vi "335 set Temp(SubVI).vi"(6 "Input (0:A)":u16(ring)=1 items=["A", "B"], 7 "Output (1:1)":u16(ring)=1 items=["1"=1, "2"=2], 8 "error in (no error)":errorcluster, 9 "Rate":dbl, 10 "Temperature":dbl, 11 "VISA Refnum in":refnum<visa-resource-name>) -> (0 "error out":errorcluster, 3 "VISA resource name out":refnum<visa-resource-name>)   [LabVIEW 2019, in "SubVI.lvlib"]
uses:
  SubVI.lvlib
  lib/Lake Shore 335/Lake Shore 335.lvlib
panel:
  out "Sensor Data 2":dbl format="%.4f"
  out "Sensor Data":dbl format="%.4f"
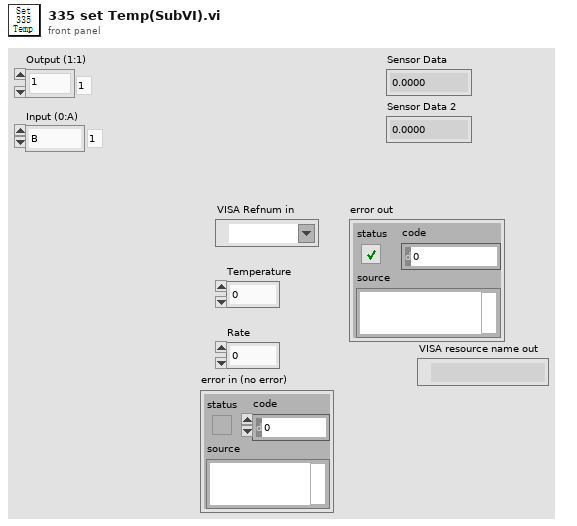
[diagram p1: front panel]
types:
  T1 = typedef "Semaphore RefNum" = refnum<k1>
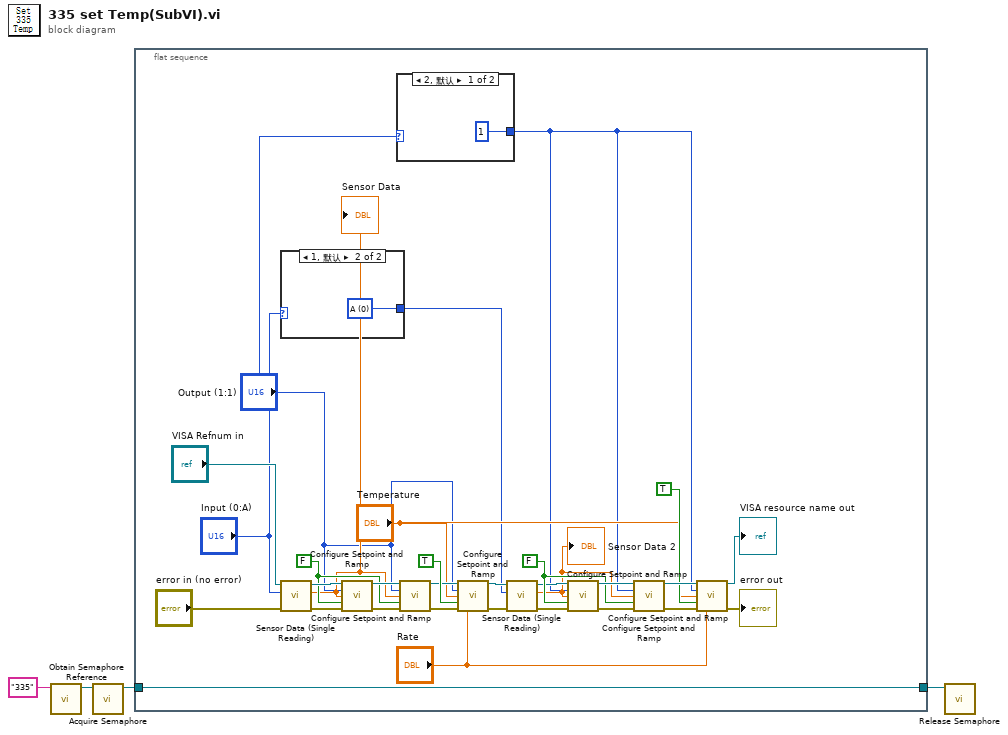
[diagram p0: block diagram]
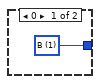
[diagram p2: hidden frame]
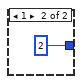
[diagram p3: hidden frame]
diagram:
  n1 = call <vilib>:"Obtain Semaphore Reference.vi"("name (unnamed)"="335") -> ("semaphore"=w3:T1)  [unwired: 4 in, 2 out]
  n2 = call <vilib>:"Acquire Semaphore.vi"("semaphore"=w3) -> ("semaphore out"=w2:T1)  [unwired: 4 in, 2 out]
  n3 = flat-sequence {
    tunnel: w2 -> [w30]
    tunnel: [w30] -> w1
    frame #0 {
      w17 = FALSE ("Enable Setpoint Ramping (F: Off)")
      w25 = FALSE ("Enable Setpoint Ramping (F: Off)")
      n4 = case shown="1, 默认" "Input (0:A)" {
        tunnel: [w36 w37] -> w6
        frame 0 {
          w36 = u16 1 items=["A", "B"] ("Input (0:A)")
        }
        frame 1, Default {
          w37 = u16 0 items=["A", "B"] ("Input (0:A)")
        }
      }
      n5 = call "Sensor Data (Single Reading).vi"("error in (no error)"="error in (no error)", "Input (0:A)"="Input (0:A)", "VISA resource name"="VISA Refnum in") -> ("error out"=w31:errorcluster, "Sensor Data"=w24:dbl, "VISA resource name out"=w34:refnum<visa-resource-name>)  [unwired: 6 in]
      "Sensor Data" <- w24
      n6 = call "Configure Setpoint and Ramp.vi"("VISA resource name"=w34, "Output's Control Loop (1:1)"="Output (1:1)", "Setpoint (0.0000)"=w24, "Enable Setpoint Ramping (F: Off)"=w25, "error in (no error)"=w31) -> ("VISA resource name out"=w27:refnum<visa-resource-name>, "error out"=w29:errorcluster)  [unwired: 9 in]
      n7 = case shown="2, 默认" "Output (1:1)" {
        tunnel: [1 2] -> w8
        frame 2, Default {
        }
        frame 1 {
        }
      }
      n8 = call "Configure Setpoint and Ramp.vi"("VISA resource name"=w27, "Output's Control Loop (1:1)"="Output (1:1)", "Setpoint (0.0000)"=w24, "Enable Setpoint Ramping (F: Off)"=w25, "error in (no error)"=w29) -> ("VISA resource name out"=w26:refnum<visa-resource-name>, "error out"=w28:errorcluster)  [unwired: 9 in]
      n9 = call "Configure Setpoint and Ramp.vi"("VISA resource name"=w26, "Output's Control Loop (1:1)"="Output (1:1)", "Setpoint (0.0000)"="Temperature", "Enable Setpoint Ramping (F: Off)"=TRUE, "error in (no error)"=w28, "Ramp Rate (0.0)"="Rate") -> ("VISA resource name out"=w16:refnum<visa-resource-name>, "error out"=w14:errorcluster)  [unwired: 8 in]
      n10 = call "Sensor Data (Single Reading).vi"("error in (no error)"=w14, "Input (0:A)"=w6, "VISA resource name"=w16) -> ("error out"=w13:errorcluster, "Sensor Data"=w12:dbl, "VISA resource name out"=w15:refnum<visa-resource-name>)  [unwired: 6 in]
      "Sensor Data 2" <- w12
      n11 = call "Configure Setpoint and Ramp.vi"("VISA resource name"=w15, "Output's Control Loop (1:1)"=w8, "Setpoint (0.0000)"=w12, "Enable Setpoint Ramping (F: Off)"=w17, "error in (no error)"=w13) -> ("VISA resource name out"=w23:refnum<visa-resource-name>, "error out"=w18:errorcluster)  [unwired: 9 in]
      n12 = call "Configure Setpoint and Ramp.vi"("VISA resource name"=w23, "Output's Control Loop (1:1)"=w8, "Setpoint (0.0000)"=w12, "Enable Setpoint Ramping (F: Off)"=w17, "error in (no error)"=w18) -> ("VISA resource name out"=w22:refnum<visa-resource-name>, "error out"=w19:errorcluster)  [unwired: 9 in]
      n13 = call "Configure Setpoint and Ramp.vi"("VISA resource name"=w22, "Output's Control Loop (1:1)"=w8, "Setpoint (0.0000)"="Temperature", "Enable Setpoint Ramping (F: Off)"=TRUE, "error in (no error)"=w19, "Ramp Rate (0.0)"="Rate") -> ("VISA resource name out"=→"VISA resource name out":refnum<visa-resource-name>, "error out"=→"error out":errorcluster)  [unwired: 8 in]
    }
  }
  n14 = call <vilib>:"Release Semaphore.vi"("semaphore"=w1) -> ()  [unwired: 5 in, 2 out]
